vi "Scan Multi Bias (With Setpoint_&_Bias_Control).vi"() -> ()   [LabVIEW 2024]
doc: "This example performs multiple image scans, increasing the bias voltage after each scan.\n\n- Nanonis Programming Interface -"
uses:
  <userlib>/Nanonis Prog Interface V5/Nanonis Prog Interface.lvlib
panel:
  in  "Setpoint":sgl[](array[numeric])=[0.0, 0.0]
  in  "Bias":sgl[](array[numeric])=[0.0, 0.0]
  in  "DISABLES DOWN SCAN":bool=TRUE
  in  "Avoid zero threshold (V)":dbl=0.004999999888241291 format="%#_13g"
  in  "Pre-scan time [ms]":dbl
  in  "Auto save":bool
  in  "Series Name":string="ScanMultiBias_" caption="Serie name"
  out "Scan":u8 caption="Current scan"
  in  "Number of scans":u8=5
  # "e"
  # "Performs multiple image scans, allowing for the fine tunning of the voltage and current during each scan."
  # "Set to 0.05M to go from -100 mV to 100 mV"
  # "Change Bias(V) Based on iteration of scan"
  # "Change Setpoint(A) Based on iteration of scan"
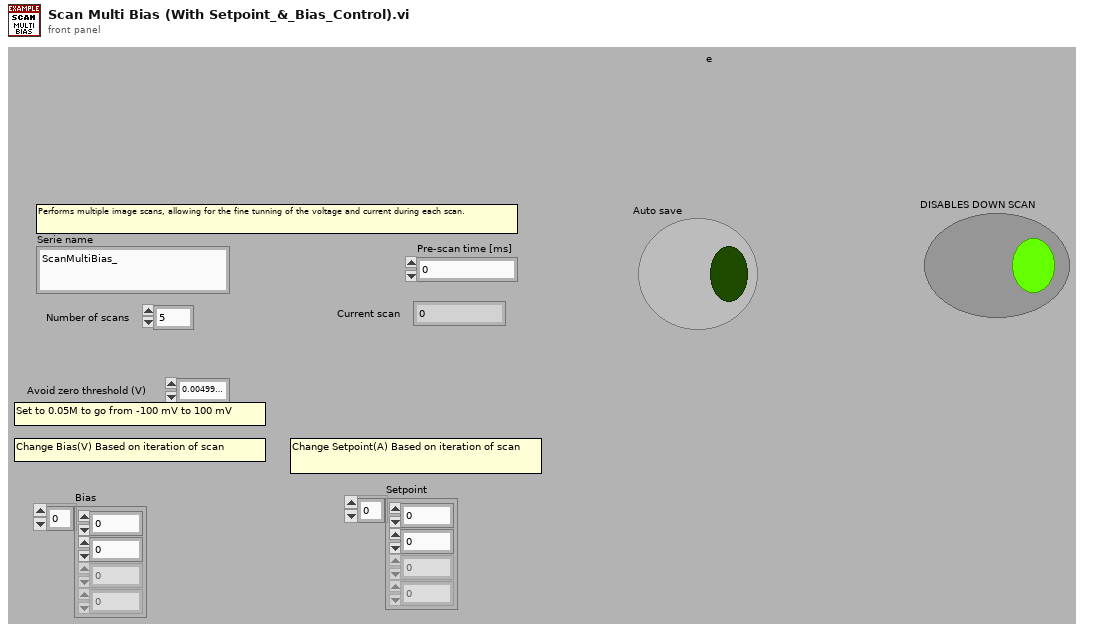
[diagram p1: front panel]
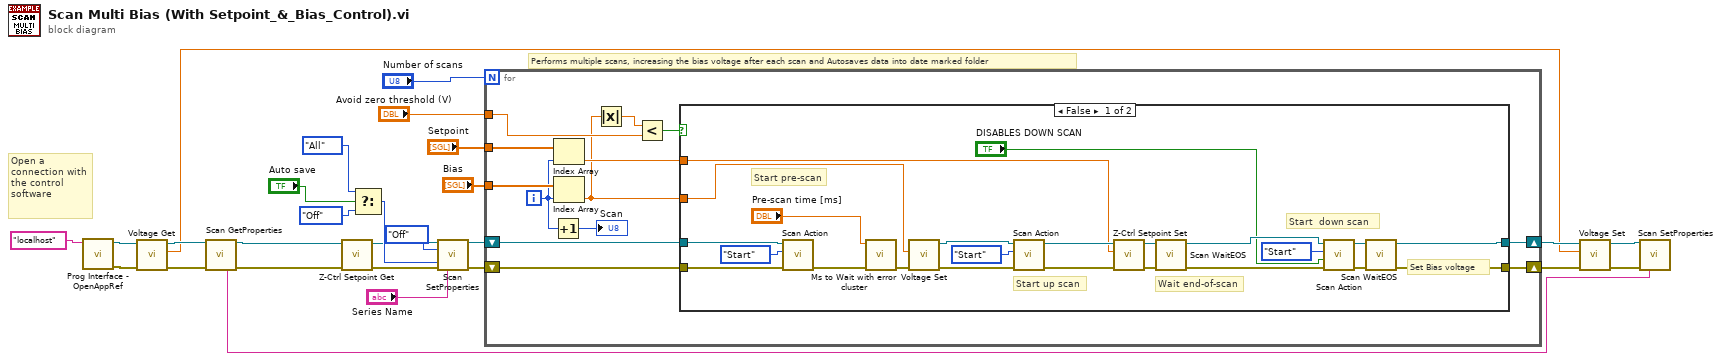
[diagram p0: block diagram]
diagram:
  # "Open a connection with the control\nsoftware"
  # "Performs multiple scans, increasing the bias voltage after each scan and Autosaves data into date marked folder"
  n1 = call <userlib>:"Prog Interface - OpenAppRef.vi"("Machine name (local machine IP)"="localhost" ("Machine name (localhost)")) -> ("Error out"=w27:errorcluster, "Application reference"=w18:refnum<vi>)  [unwired: 5 in]
  n2 = call <userlib>:"Voltage Get.vi"("error in (no error)"=w27, "Application ref in"=w18) -> ("error out"=w13:errorcluster, "Bias (V)"=w3:sgl, "Application ref out"=w14:refnum<vi>)  [unwired: 7 in]
  n3 = call <userlib>:"Scan GetProperties.vi"("Application ref in"=w14, "Error in (no error)"=w13) -> ("Application ref out"=w9:refnum<vi>, "Serie name"=w12:string, "Error out"=w10:errorcluster)  [unwired: 6 in, 5 out]
  n4 = call <userlib>:"Z-Ctrl Setpoint Get.vi"("error in (no error)"=w10, "Application ref in"=w9) -> ("error out"=w7:errorcluster, "Application ref out"=w8:refnum<vi>)  [unwired: 6 in, 1 out]
  n5 = Select(t=enum16{"No change", "All", "Next", "Off"}."All" ("Auto save"), s="Auto save", f=enum16{"No change", "All", "Next", "Off"}."Off" ("Auto save")) -> (s? t:f=w19:enum16{"No change", "All", "Next", "Off"})
  n6 = call <userlib>:"Scan SetProperties.vi"("Application ref in"=w8, "Continuous scan"=enum16{"No change", "On", "Off"}."Off", "Auto save"=w19, "Error in (no error)"=w7, "Serie name"="Series Name") -> ("Application ref out"=w17:refnum<vi>, "Error out"=w25:errorcluster)  [unwired: 9 in]
  n7 = for {
    N: "Number of scans" -> [_]
    shift-right: [w35] -> w15
    shift-left: w25 -> [w40]
    shift-right: [w36] -> w16
    shift-left: w17 -> [w39]
    tunnel: "Avoid zero threshold (V)" -> [w34]
    tunnel: "Setpoint" -> [w33]
    tunnel: "Bias" -> [w30]
    i -> [w29]
    n8 = Increment(x=w29) -> (x+1=→"Scan":i32)
    n9 = Index Array(array=w33, index=w29) -> (element=w32:sgl)
    n10 = Index Array(array=w30, index=w29) -> (element=w28:sgl)
    n11 = Absolute Value(x=w28) -> (abs(x)=w38:sgl)
    n12 = Less?(x=w38, y=w34) -> (x < y?=w37:bool)
    n13 = case shown="False" w37 {
      tunnel: w40 -> [w63 w64]
      tunnel: w28 -> [w41 _]
      tunnel: w39 -> [w61 w65]
      tunnel: [w45 w65] -> w36
      tunnel: [w46 w64] -> w35
      tunnel: w32 -> [w47 _]
      frame False {
        # "Start  down scan"
        # "Start up scan"
        # "Set Bias voltage"
        # "Wait end-of-scan"
        # "Start pre-scan"
        n14 = call <userlib>:"Scan Action.vi"("error in (no error)"=w63, "Scan action (Start)"=enum16{"Start", "Stop", "Pause", "Resume"}."Start" ("Scan action"), "Application ref in"=w61) -> ("error out"=w59:errorcluster)  [unwired: 6 in, 1 out]
        n15 = call <userlib>:"Ms to Wait with error cluster.vi"("error in (no error)"=w59, "milliseconds to wait"="Pre-scan time [ms]") -> ("error out"=w42:errorcluster)  [unwired: 4 in, 1 out]
        n16 = call <userlib>:"Voltage Set.vi"("Error in (no error)"=w42, "Bias (V)"=w41) -> ("Error out"=w43:errorcluster, "Application ref out"=w44:refnum<vi>)  [unwired: 8 in]
        n17 = call <userlib>:"Scan Action.vi"("error in (no error)"=w43, "Scan action (Start)"=enum16{"Start", "Stop", "Pause", "Resume"}."Start" ("Scan action"), "Application ref in"=w44) -> ("error out"=w51:errorcluster, "Application ref out"=w48:refnum<vi>)  [unwired: 6 in]
        n18 = call <userlib>:"Z-Ctrl Setpoint Set.vi"("error in (no error)"=w51, "Z Controller setpoint"=w47, "Application ref in"=w48) -> ("error out"=w50:errorcluster, "Application ref out"=w49:refnum<vi>)  [unwired: 7 in]
        n19 = call <userlib>:"Scan WaitEOS.vi"("error in (no error)"=w50, "Application ref in"=w49) -> ("error out"=w56:errorcluster, "Application ref out"=w57:refnum<vi>)  [unwired: 5 in, 2 out]
        n20 = call <userlib>:"Scan Action.vi"("error in (no error)"=w56, "Direction: up/down (T=up)"="DISABLES DOWN SCAN", "Scan action (Start)"=enum16{"Start", "Stop", "Pause", "Resume"}."Start", "Application ref in"=w57) -> ("error out"=w54:errorcluster, "Application ref out"=w53:refnum<vi>)  [unwired: 5 in]
        n21 = call <userlib>:"Scan WaitEOS.vi"("error in (no error)"=w54, "Application ref in"=w53) -> ("error out"=w46:errorcluster, "Application ref out"=w45:refnum<vi>)  [unwired: 5 in, 2 out]
      }
      frame True {
      }
    }
  }
  n22 = call <userlib>:"Voltage Set.vi"("Error in (no error)"=w15, "Bias (V)"=w3, "Application ref in"=w16) -> ("Error out"=w5:errorcluster, "Application ref out"=w4:refnum<vi>)  [unwired: 7 in]
  n23 = call <userlib>:"Scan SetProperties.vi"("Application ref in"=w4, "Error in (no error)"=w5, "Serie name"=w12) -> ()  [unwired: 11 in, 2 out]
